vi "4155C QSCV.vi"(0 "VISA resource name in":refnum<visa-resource-name>="GPIB0::14::INSTR", 1 "Timings":T2={"hold time (sec)"=0.0, "delay time (sec)"=0.0, "Step Time (0 disables)"=0.0, "C-Step"=0.1, "CInt"=0.1, "IInt"=0.1} {"IInt" min=0.01 max=10.0 format="%.2f"; "CInt" min=0.01 max=10.0 format="%.2f"; "C-Step" min=0.01 max=10.0 format="%.2f"; "Step Time (0 disables)" min=0.0 format="%.2f"; "delay time (sec)" min=0.0 format="%.4f"; "hold time (sec)" min=0.0 format="%.4f"}, 2 "Drain":T4={"Drain voltage"=0.0, "Drain Compliance"=0.0001, "Range mode"=0, "Range"=6} {"Range" max=11 scale=0.0..11.0; "Range mode" items=["Auto", "Limited", "Fixed"]; "Drain Compliance" min=0.0 max=0.1 format="%^.2e"; "Drain voltage" min=-100.0 max=100.0 format="%^.4e"}, 3 "Gate":T3={"Gate Start"=0.0, "Gate Stop"=2.0, "Gate Step"=1.0, "Gate Compliance"=0.0001, "Range mode"=0, "Range"=6} {"Range" max=11 scale=0.0..11.0; "Range mode" items=["Auto", "Limited", "Fixed"]; "Gate Compliance" min=0.0 max=0.1 format="%^.2e"; "Gate Step" min=-100.0 max=100.0 format="%^.4e"; "Gate Stop" min=-100.0 max=100.0 format="%^.4e"; "Gate Start" min=-100.0 max=100.0 format="%^.4e"}, 4 "Panel Controls":T1={"Emergency Stop"=refnum, "CapGraph Max"=1e-05, "Text/Graph (text=false)"=FALSE} {"CapGraph Max" format="%.2e"}, 5 "error in (no error)":errorcluster, 6 "sweep mode":u16(ring) items=["Single", "Double"]) -> (14 "VISA Resource Name out":refnum<visa-resource-name>, 15 "VG":dbl[](array[numeric]) format="%.2f", 16 "Cap":dbl[](array[numeric]) format="%.2f", 17 "Leak":dbl[](array[numeric]) format="%.2f", 18 "Number of points":i32=1, 19 "error out":errorcluster)   [LabVIEW 2016]
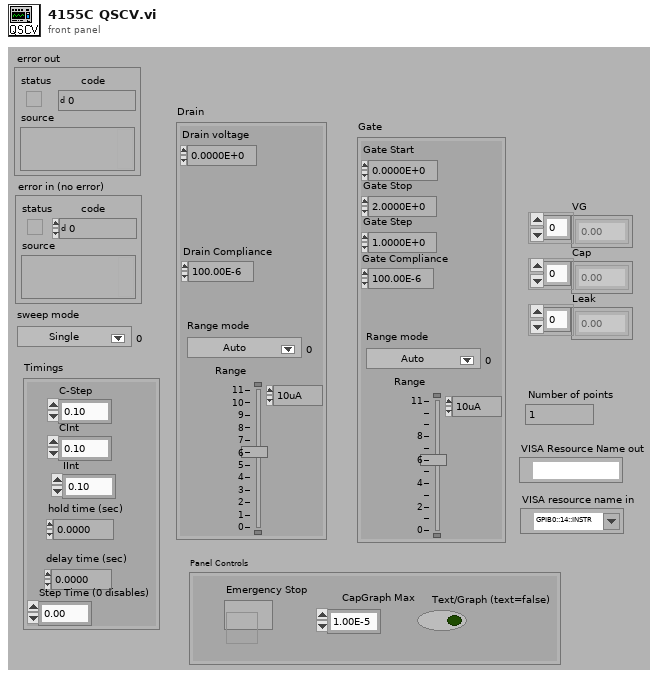
[diagram p1: front panel]
types:
  T1 = cluster{"Emergency Stop":refnum<vi>, "CapGraph Max":dbl, "Text/Graph (text=false)":bool}
  T2 = cluster{"hold time (sec)":dbl, "delay time (sec)":dbl, "Step Time (0 disables)":dbl, "C-Step":dbl, "CInt":dbl, "IInt":dbl}
  T3 = cluster{"Gate Start":dbl, "Gate Stop":dbl, "Gate Step":dbl, "Gate Compliance":dbl, "Range mode":u16, "Range":u8}
  T4 = cluster{"Drain voltage":dbl, "Drain Compliance":dbl, "Range mode":u16, "Range":u8}
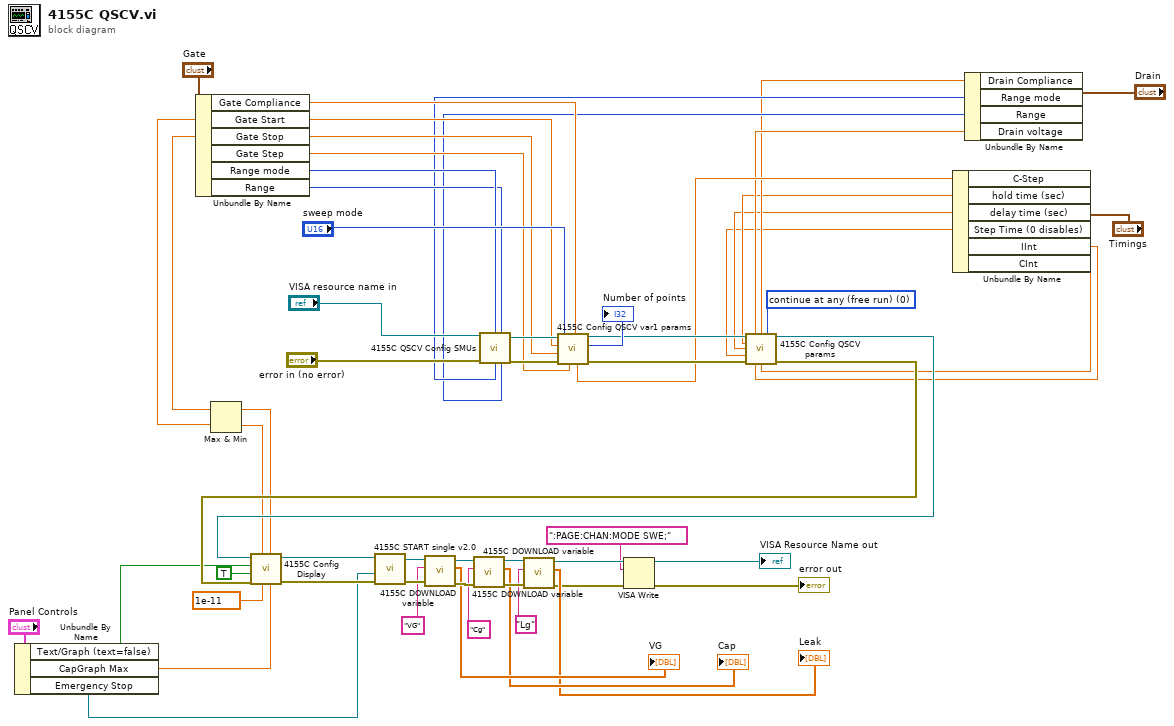
[diagram p0: block diagram]
diagram:
  w6 = u8 0 items=["continue at any (free run)", "stop at any abnorm", "stop at compliance"] ("stop condition (free run:0)")
  n1 = Unbundle By Name("Panel Controls") -> ("Text/Graph (text=false)"=w23:bool, "CapGraph Max"=w7:dbl, "Emergency Stop"=w25:refnum<vi>)
  n2 = Unbundle By Name("Gate") -> ("Gate Compliance"=w41:dbl, "Gate Start"=w29:dbl, "Gate Stop"=w28:dbl, "Gate Step"=w40:dbl, "Range mode"=w22:u16, "Range"=w21:u8)
  n3 = Max & Min(x=w28, y=w29) -> (max(x,y)=w26:dbl, min(x,y)=w27:dbl)
  n4 = Unbundle By Name("Timings") -> ("C-Step"=w15:dbl, "hold time (sec)"=w12:dbl, "delay time (sec)"=w11:dbl, "Step Time (0 disables)"=w10:dbl, "IInt"=w9:dbl, "CInt"=w8:dbl)
  n5 = Unbundle By Name("Drain") -> ("Drain Compliance"=w13:dbl, "Range mode"=w20:u16, "Range"=w19:u8, "Drain voltage"=w14:dbl)
  n6 = call "4155C QSCV Config SMUs.vi"("VISA resource name in"="VISA resource name in", "Gate mode"=w22, "Gate Range"=w21, "error in (no error)"="error in (no error)", "Source/drain mode"=w20, "Source/drain Range"=w19) -> ("VISA Resource Name out"=w47:refnum<visa-resource-name>, "error out"=w46:errorcluster)  [unwired: 8 in]
  n7 = call "4155C Config QSCV var1 params.vi"("Cap Step"=w15, "compliance"=w41, "step"=w40, "sweep mode"="sweep mode", "error in (no error)"=w46, "stop"=w28, "start"=w29, "VISA session"=w47) -> ("error out"=w16:errorcluster, "Number of points"=→"Number of points":i32, "dup VISA resource name"=w17:refnum<visa-resource-name>)  [unwired: 1 in]
  n8 = call "4155C Config QSCV params.vi"("VISA session"=w17, "Drain Voltage"=w14, "Drain Compliance"=w13, "stop condition (free run:0)"=w6, "HTIMe"=w12, "DELay"=w11, "RANGe"=w10, "error in (no error)"=w16, "I-Int"=w9, "C-Int"=w8) -> ("dup VISA resource name"=w30:refnum<visa-resource-name>, "error out"=w31:errorcluster)  [unwired: 4 in]
  n9 = call "4155C Config Display.vi"("Ymax"=w7, "Var1 Stop"=w26, "Ymin"=1e-11, "Var1 Start"=w27, "error in (no error)"=w31, "Logarithmic"=TRUE, "SPA Display"=w23, "VISA session"=w30) -> ("error out"=w32:errorcluster, "dup VISA resource name"=w33:refnum<visa-resource-name>)  [unwired: 2 in]
  n10 = call "4155C START single v2.0.vi"("error in (no error)"=w32, "Emergency Stop"=w25, "VISA resource name in"=w33) -> ("error out"=w56:errorcluster, "VISA Resource Name out"=w57:refnum<visa-resource-name>)  [unwired: 3 in]
  n11 = call "4155C DOWNLOAD variable.vi"("error in (no error)"=w56, "Variable name"="VG", "VISA resource name in"=w57) -> ("error out"=w54:errorcluster, "Output data"=→"VG":dbl[], "VISA Resource Name out"=w53:refnum<visa-resource-name>)  [unwired: 2 in]
  n12 = call "4155C DOWNLOAD variable.vi"("error in (no error)"=w54, "Variable name"="Cg", "VISA resource name in"=w53) -> ("error out"=w50:errorcluster, "Output data"=→"Cap":dbl[], "VISA Resource Name out"=w51:refnum<visa-resource-name>)  [unwired: 2 in]
  n13 = call "4155C DOWNLOAD variable.vi"("error in (no error)"=w50, "Variable name"="Lg", "VISA resource name in"=w51) -> ("error out"=w2:errorcluster, "Output data"=→"Leak":dbl[], "VISA Resource Name out"=w5:refnum<visa-resource-name>)  [unwired: 2 in]
  n14 = VISA Write(VISA resource name=w5, write buffer=":PAGE:CHAN:MODE SWE;" ("write buffer (\"\")"), error in (no error)=w2) -> (VISA resource name out=→"VISA Resource Name out":refnum<visa-resource-name>, error out=→"error out":errorcluster)  [unwired: 1 out]
